vi "KT2.vi"() -> ()   [LabVIEW 2018]
doc: "Read from custom VI temperature 10 times /seconds"
uses:
  Downloads/Global 2.vi
panel:
  out "Temperature":dbl
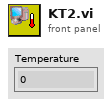
[diagram p1: front panel]
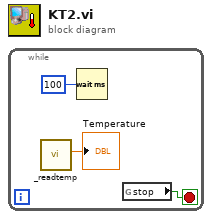
[diagram p0: block diagram]
diagram:
  n1 = while {
    stop <- w1 stop-if-true
    n2 = call "_readtemp.vi"() -> ("Temperature"=→"Temperature":dbl)  [unwired: 10 in, 1 out]
    n3 = Wait (ms)(milliseconds to wait=u32 100) -> ()  [unwired: 1 out]
    n4 = global read "Global 2.vi" "stop"() -> (w1:bool)
  }
